vi "Rising Edge (Windowed).vi"(7 "Window":u8=10, 11 "Input":bool) -> (3 "Rising Edge?":bool)   [LabVIEW 2014]
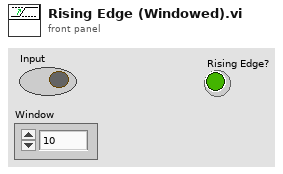
[diagram p1: front panel]
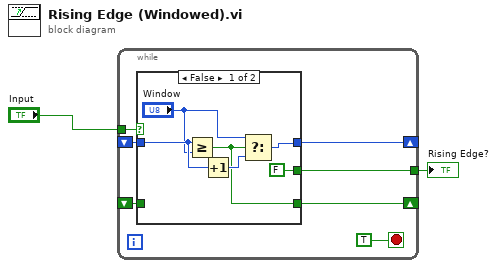
[diagram p0: block diagram]
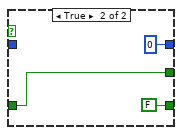
[diagram p2: hidden frame]
diagram:
  n1 = while {
    tunnel: "Input" -> [w8]
    shift-right: [w6] -> _
    shift-left: _ -> [w7]
    shift-right: [w5] -> _
    shift-left: _ -> [w4]
    tunnel: [w3] -> w2
    stop <- TRUE stop-if-true
    n2 = case shown="False" w8 {
      tunnel: w7 -> [w15 _]
      tunnel: [w13 u8 0 ("t")] -> w6
      tunnel: [w12 FALSE] -> w5
      tunnel: w4 -> [_ w16]
      tunnel: [FALSE w16] -> w3
      frame False {
        n3 = Greater Or Equal?(x=w15, y="Window") -> (x >= y?=w12:bool)
        n4 = Increment(x=w15) -> (x+1=w14:u8)
        n5 = Select(t="Window", s=w12, f=w14) -> (s? t:f=w13:u8)
      }
      frame True {
      }
    }
  }
  "Rising Edge?" <- w2
